vi "Actuation Signal.vi"(0 "On-time (ms)":u32, 1 "LINX Resource":T1, 5 "Frequency":u32, 7 "Pin Number":u8, 9 "On or Off?":bool, 11 "Error In":errorcluster) -> (4 "LINX Resource 2":T1, 15 "Error Out":errorcluster)   [LabVIEW 2017]
uses:
  <vilib>/MakerHub/LINX/Private/Type Defs/LINX Ref.ctl
  <vilib>/MakerHub/LINX/Private/Type Defs/Platform.ctl
  <vilib>/MakerHub/LINX/Private/Type Defs/Interface.ctl
  <vilib>/MakerHub/LINX/Private/Device/Type Defs/LINX Device Config.ctl
  <vilib>/MakerHub/LINX/Private/Device/Type Defs/TCP Config.ctl
  <vilib>/MakerHub/LINX/Private/Device/Type Defs/Channels.ctl
  <vilib>/MakerHub/LINX/Public/Peripherals/Digital/Digital Write 1 Chan.vi
  <vilib>/MakerHub/LINX/Public/Peripherals/Digital/Digital Write N Chans.vi
  <vilib>/MakerHub/LINX/Private/Local IO/LinxDigitalWrite.vi
  <vilib>/MakerHub/LINX/Public/Utilities/Check Channel.vi
  <vilib>/MakerHub/LINX/Private/Utilties/Generate Error.vi
  <vilib>/MakerHub/LINX/LMH-LINX.lvlib
  <vilib>/MakerHub/LINX/Private/Device/Device.lvlib
panel:
  in  "DC or AC?":bool
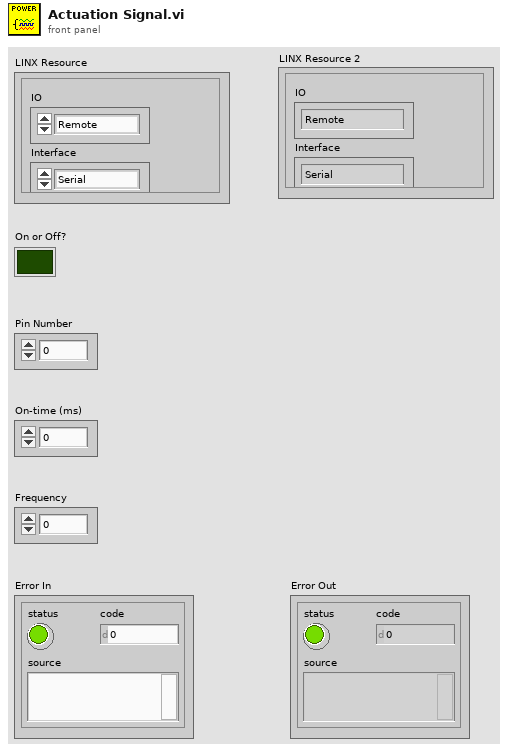
[diagram p1: front panel]
types:
  T1 = typedef "LMH-LINX.lvlib/LINX Ref.ctl" = cluster{"IO":T2, "Interface":T3, "LINX Device Config":T4}
  T2 = typedef "LMH-LINX.lvlib/Platform.ctl" = enum16{"Remote", "Local"}
  T3 = typedef "LMH-LINX.lvlib/Interface.ctl" = enum16{"Serial", "TCP"}
  T4 = typedef "LMH-LINX.lvlib/Device.lvlib/LINX Device Config.ctl" = cluster{"Interface":T3, "COM Port":refnum<visa-resource-name>, "TCP Configuration":T5, "Device Family":u8, "Device ID":u8, "Device Name":string, "TCP Ref":refnum<k5>, "Channels":T6}
  T5 = typedef "LMH-LINX.lvlib/Device.lvlib/TCP Config.ctl" = cluster{"IP Address":string, "Port":u16}
  T6 = typedef "LMH-LINX.lvlib/Channels.ctl" = cluster{"DI":u8[], "DO":u8[], "AI":u8[], "AO":u8[], "PWM":u8[], "QE":u8[], "UART":u8[], "I2C 2":u8[], "SPI":u8[], "CAN":u8[], "Servo":u8[], "AI Ref (V)":dbl, "AI Resolution (Bits)":u8, "AO Ref (V)":dbl, "AO Resolution (Bits)":u8}
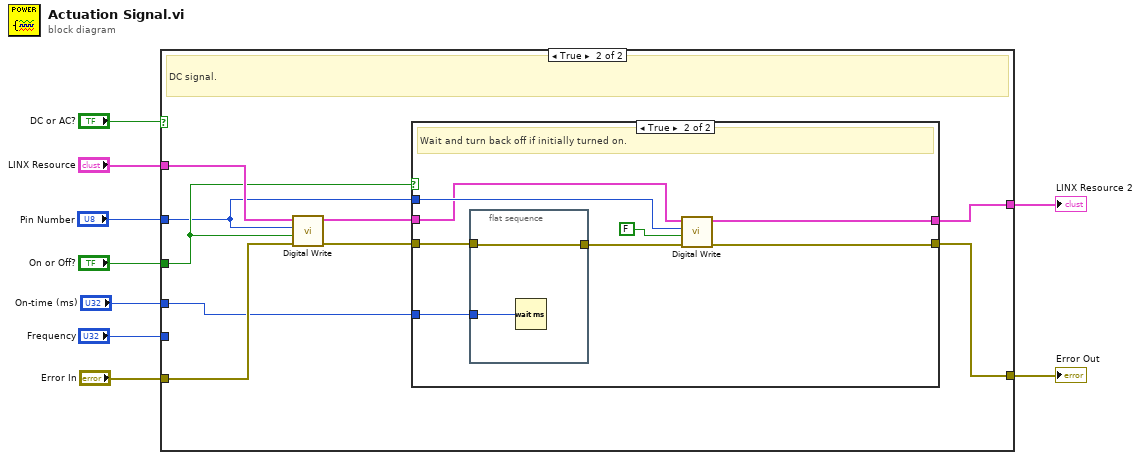
[diagram p0: block diagram]
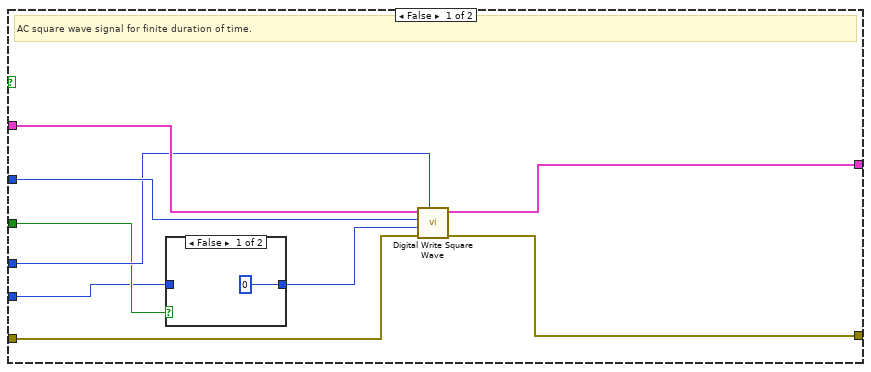
[diagram p2: hidden frame]
diagram:
  n1 = case shown="True" "DC or AC?" {
    tunnel: "Error In" -> [w16 w29]
    tunnel: "On-time (ms)" -> [w15 w27]
    tunnel: "Frequency" -> [w13 _]
    tunnel: "LINX Resource" -> [w18 w28]
    tunnel: "On or Off?" -> [w14 w24]
    tunnel: "Pin Number" -> [w17 w23]
    tunnel: [w11 w22] -> w2
    tunnel: [w10 w21] -> w1
    frame False {
      # "AC square wave signal for finite duration of time."
      n2 = case shown="False" w14 {
        tunnel: w13 -> [_ w20]
        tunnel: [u32 0 ("Frequency") w20] -> w12
        frame False {
        }
        frame True {
        }
      }
      n3 = call <vilib>:"Digital Write Square Wave.vi"("Duration (ms)"=w15, "Error In"=w16, "Frequency (Hz)"=w12, "Channel"=w17, "LINX Resource"=w18) -> ("Error Out"=w11:errorcluster, "LINX Resource"=w10:T1)  [unwired: 5 in]
    }
    frame True {
      # "DC signal."
      n4 = call-poly <vilib>:"Digital Write.vi"("Error In"=w29, "Output Value"=w24, "DO Channel"=w23, "LINX Resource"=w28) -> ("Error Out"=w26:errorcluster, "LINX Resource"=w25:T1)  [unwired: 6 in]
      n5 = case shown="True" w24 {
        tunnel: w27 -> [_ w39]
        tunnel: w26 -> [w31 w38]
        tunnel: w25 -> [w30 w35]
        tunnel: w23 -> [_ w36]
        tunnel: [w31 w33] -> w22
        tunnel: [w30 w32] -> w21
        frame False {
          # "No action required if turning off."
        }
        frame True {
          # "Wait and turn back off if initially turned on."
          n6 = flat-sequence {
            tunnel: w39 -> [w41]
            tunnel: w38 -> [w40]
            tunnel: [w40] -> w37
            frame #0 {
              n7 = Wait (ms)(milliseconds to wait=w41) -> ()  [unwired: 1 out]
            }
          }
          n8 = call-poly <vilib>:"Digital Write.vi"("Error In"=w37, "Output Value"=FALSE, "DO Channel"=w36, "LINX Resource"=w35) -> ("Error Out"=w33:errorcluster, "LINX Resource"=w32:T1)  [unwired: 6 in]
        }
      }
    }
  }
  "Error Out" <- w2
  "LINX Resource 2" <- w1
